vi "CMD_Loop.vi"() -> ()   [LabVIEW 2020, in "SubCMD_CMD.lvlib"]
uses:
  SubCMD_CMD.lvlib
  Cluster_CMD_CMD_Data.ctl
  ENUM_CMD_State.ctl
  ENUM_CMD_Action.ctl
  Global_CMD_CMD_Data In.vi
  Utility/Global_STOP.vi
  Global_CMD_Data Out.vi
panel:
  out "Input Data":T1
  out "Cycle Time (S)":dbl format="%.3g"
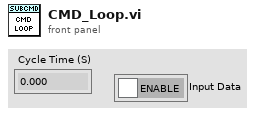
[diagram p1: front panel]
types:
  T1 = typedef "SubCMD_CMD.lvlib/Cluster_CMD_CMD_Data.ctl" = cluster{"ENABLE":bool}
  T2 = typedef "SubCMD_CMD.lvlib/ENUM_CMD_State.ctl" = enum16{"Startup", "Idle", "Shutdown"}
  T3 = typedef "SubCMD_CMD.lvlib/ENUM_CMD_Action.ctl" = enum16{"No Action", "Reset Time", "Reset All", "Action A", "Action B"}
  T4 = cluster{"State":T2, "Previous State":T2, "Current Time":timestamp, "Previous Time":timestamp, "Start Time":timestamp, "Target Time (ms)":u32, "Cycle Time(S)":dbl, "CMD Input":T1, "Output DBL":dbl}
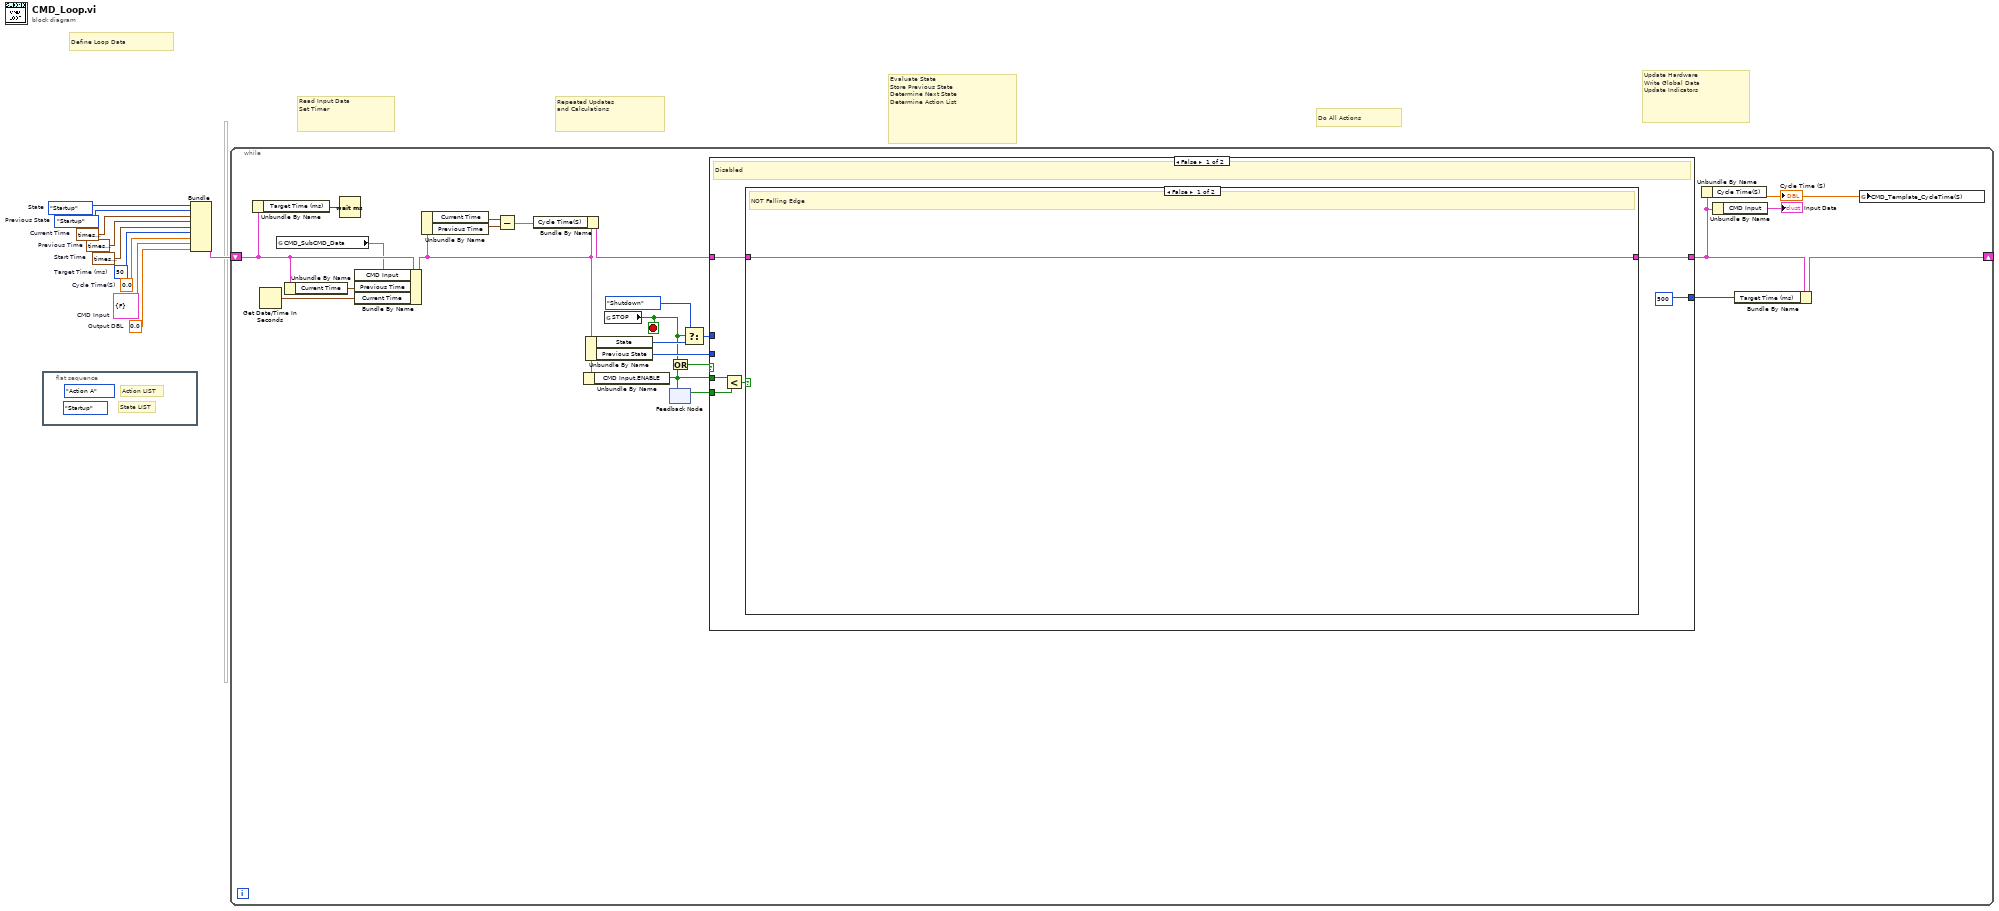
[diagram p0: block diagram]
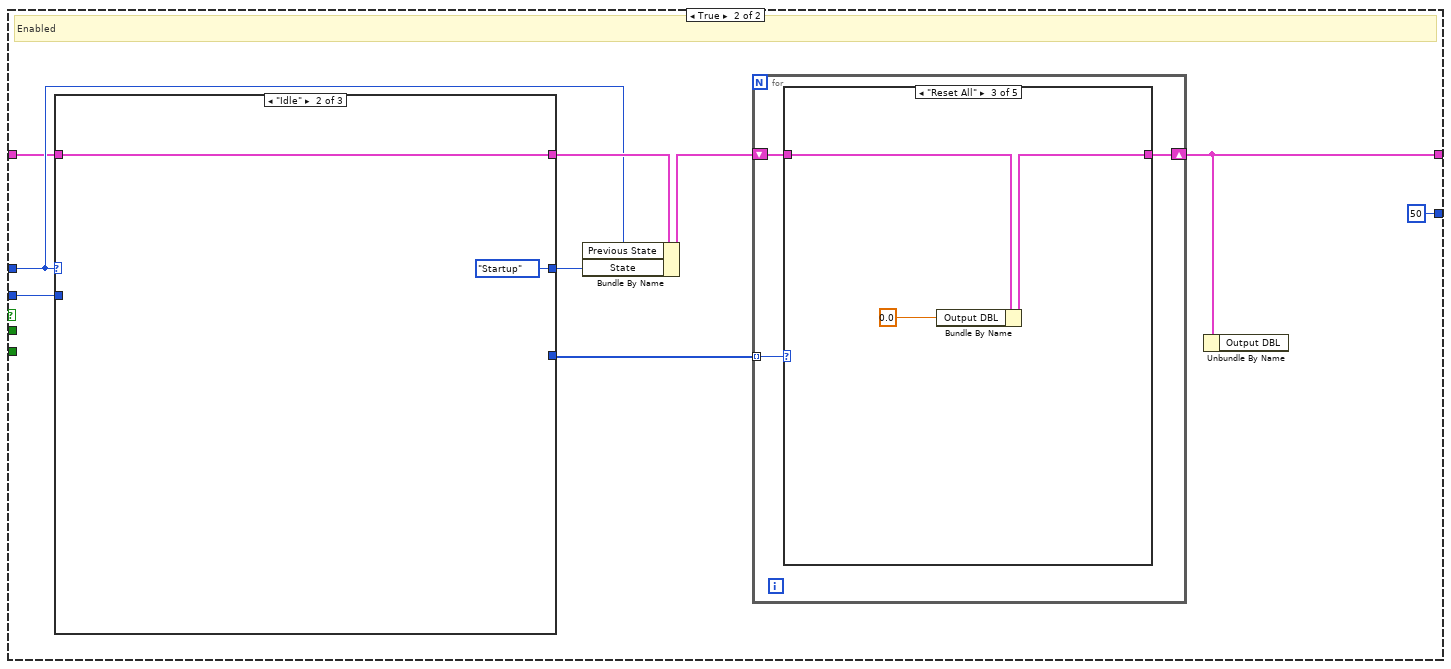
[diagram p3: hidden frame]
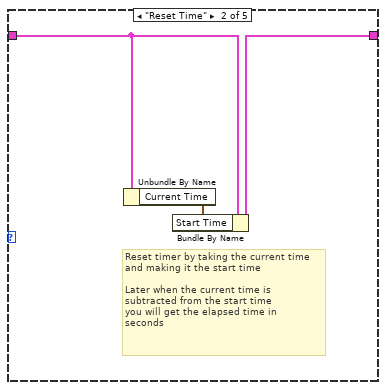
[diagram p5: hidden frame]
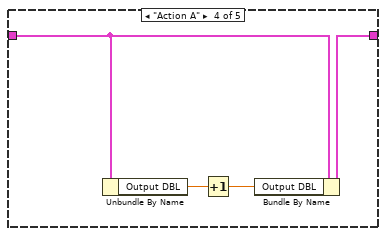
[diagram p6: hidden frame]
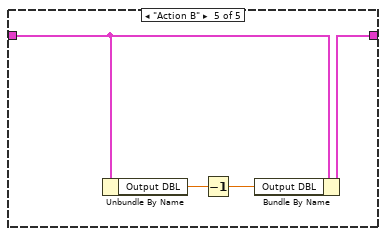
[diagram p7: hidden frame]
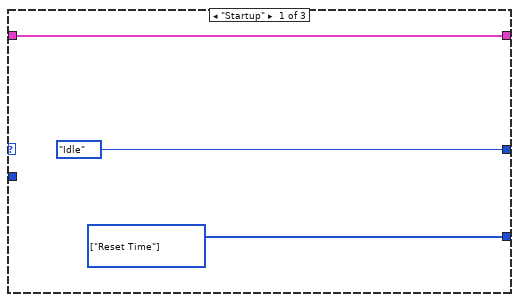
[diagram p8: hidden frame]
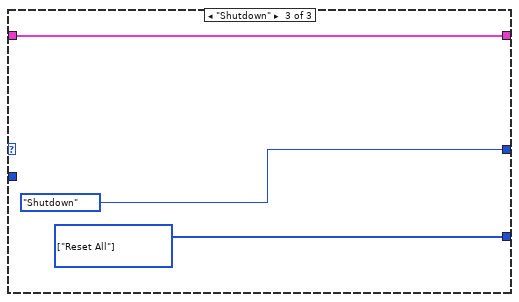
[diagram p9: hidden frame]
diagram:
  w1 = 0.0  # Cycle Time(S)
  w2 = ENUM_CMD_State."Startup"  # Previous State
  w3 = timestamp(0 s since 1904-01-01)  # Previous Time
  w4 = u32 50  # Target Time (ms)
  w5 = 0.0  # Output DBL
  w6 = T1 {"ENABLE"=FALSE}  # CMD Input
  w7 = timestamp(0 s since 1904-01-01)  # Start Time
  w8 = timestamp(0 s since 1904-01-01)  # Current Time
  w9 = ENUM_CMD_State."Startup"  # State
  # "Define Loop Data"
  # "Repeated Updates\nand Calculations"
  # "Read Input Data\nSet Timer"
  # "Evaluate State\nStore Previous State\nDetermine Next State\nDetermine Action List"
  # "Do All Actions"
  # "Update Hardware\nWrite Global Data\nUpdate Indicators"
  n1 = flat-sequence {
    frame #0 {
      (unwired) ENUM_CMD_State."Startup" ("State")
      (unwired) ENUM_CMD_Action."Action A" ("Action")
      # "State LIST"
      # "Action LIST"
    }
  }
  n2 = Bundle("State"=w9, "Previous State"=w2, "Current Time"=w8, "Previous Time"=w3, "Start Time"=w7, "Target Time (ms)"=w4, "Cycle Time(S)"=w1, "CMD Input"=w6, "Output DBL"=w5) -> (w10:T4)  [unwired: 1 in]
  n3 = while {
    shift-right: [w14] -> _
    shift-left: w10 -> [w30]
    stop <- w17 stop-if-true
    n4 = Unbundle By Name(w30) -> ("Target Time (ms)"=w32:u32)
    n5 = Get Date/Time In Seconds() -> (seconds since 1Jan1904=w33:timestamp)
    n6 = global read "Global_CMD_CMD_Data In.vi" "CMD_SubCMD_Data"() -> (w29:T1)
    n7 = Unbundle By Name(w30) -> ("Current Time"=w31:timestamp)
    n8 = Wait (ms)(milliseconds to wait=w32) -> ()  [unwired: 1 out]
    n9 = Bundle By Name(cluster=w30, "CMD Input"=w29, "Previous Time"=w31, "Current Time"=w33) -> (w18:T4)
    n10 = Unbundle By Name(w18) -> ("Current Time"=w23:timestamp, "Previous Time"=w24:timestamp)
    n11 = Subtract(x=w23, y=w24) -> (x-y=w22:dbl)
    n12 = Bundle By Name(cluster=w18, "Cycle Time(S)"=w22) -> (w19:T4)
    n13 = Unbundle By Name(w18) -> ("CMD Input.ENABLE"=w12:bool)
    n14 = Unbundle By Name(w18) -> ("State"=w27:T2, "Previous State"=w26:T2)
    n15 = global read "Global_STOP.vi" "STOP"() -> (w17:bool)
    n16 = feedback-in #1(w12) -> ()
    n17 = feedback #1() -> (w11:bool)  [unwired: 1 in]
    n18 = Or(x=w17, y=w12) -> (x .or. y?=w16:bool)
    n19 = Select(t=ENUM_CMD_State."Shutdown" ("State"), s=w17, f=w27) -> (s? t:f=w25:T2)
    n20 = case shown="False" w16 {
      tunnel: [w34 w50] -> w15
      tunnel: w26 -> [_ w46]
      tunnel: w25 -> [_ w45]
      tunnel: w19 -> [w35 w44]
      tunnel: [u32 500 ("Target Time (ms)") u32 50 ("Target Time (ms)")] -> w13
      tunnel: w12 -> [w38 _]
      tunnel: w11 -> [w37 _]
      frame False {
        # "Disabled"
        n21 = Less?(x=w38, y=w37) -> (x < y?=w36:bool)
        n22 = case shown="False" w36 {
          tunnel: w35 -> [w40 w41]
          tunnel: [w40 w41] -> w34
          frame False {
            # "NOT Falling Edge"
          }
          frame True {
            # "Falling Edge"
          }
        }
      }
      frame True {
        # "Enabled"
        n23 = case shown="\"Idle\"" w45 {
          tunnel: w44 -> [w71 w73 w76]
          tunnel: [w71 w73 w76] -> w48
          tunnel: [ENUM_CMD_State."Idle" ("State") ENUM_CMD_State."Startup" ("State") ENUM_CMD_State."Shutdown" ("State")] -> w47
          tunnel: [w70 _ w74] -> w43
          tunnel: w46 -> [_ _ _]
          frame "Startup" {
            w70 = T3[] [enum."Reset Time"] items=["No Action", "Reset Time", "Reset All", "Action A", "Action B"] ("Actions")
          }
          frame "Idle" {
          }
          frame "Shutdown" {
            w74 = T3[] [enum."Reset All"] items=["No Action", "Reset Time", "Reset All", "Action A", "Action B"] ("Actions")
          }
        }
        n24 = Bundle By Name(cluster=w48, "Previous State"=w45, "State"=w47) -> (w49:T4)
        n25 = for {
          tunnel: w43 -> [w53] mode=indexing
          shift-right: [w52] -> w50
          shift-left: w49 -> [w51]
          n26 = case shown="\"Reset All\"" w53 {
            tunnel: w51 -> [w54 w57 w60 w63 w67]
            tunnel: [w54 w56 w59 w62 w66] -> w52
            frame "No Action" {
            }
            frame "Reset Time" {
              # "Reset timer by taking the current time\nand making it the start time\n\nLater when the current time is \nsubtracted from the start time\nyou will get the elapsed time in \nseconds"
              n27 = Unbundle By Name(w57) -> ("Current Time"=w55:timestamp)
              n28 = Bundle By Name(cluster=w57, "Start Time"=w55) -> (w56:T4)
            }
            frame "Reset All" {
              n29 = Bundle By Name(cluster=w60, "Output DBL"=0.0 ("FG Write Value")) -> (w59:T4)
            }
            frame "Action A" {
              n30 = Unbundle By Name(w63) -> ("Output DBL"=w64:dbl)
              n31 = Increment(x=w64) -> (x+1=w61:dbl)
              n32 = Bundle By Name(cluster=w63, "Output DBL"=w61) -> (w62:T4)
            }
            frame "Action B" {
              n33 = Unbundle By Name(w67) -> ("Output DBL"=w68:dbl)
              n34 = Decrement(x=w68) -> (x-1=w65:dbl)
              n35 = Bundle By Name(cluster=w67, "Output DBL"=w65) -> (w66:T4)
            }
          }
        }
        n36 = Unbundle By Name(w50) -> ()  [unwired: 1 out]
      }
    }
    n37 = Unbundle By Name(w15) -> ("Cycle Time(S)"=w20:dbl)
    "Cycle Time (S)" <- w20
    n38 = Unbundle By Name(w15) -> ("CMD Input"=→"Input Data":T1)
    n39 = Bundle By Name(cluster=w15, "Target Time (ms)"=w13) -> (w14:T4)
    n40 = global write "Global_CMD_Data Out.vi" "CMD_Template_CycleTime(S)"(w20) -> ()
  }
